vi "菜单-导出py.vi"(8 "error in (no error)":errorcluster caption="错误输入（无错误）", 11 "程序响应 输入":refnum<class "程序响应.lvclass">) -> (0 "error out":errorcluster caption="错误输出", 3 "程序响应 输出":refnum<class "程序响应.lvclass">)   [LabVIEW 2018, in "程序响应.lvlib" / "程序响应.lvclass"]
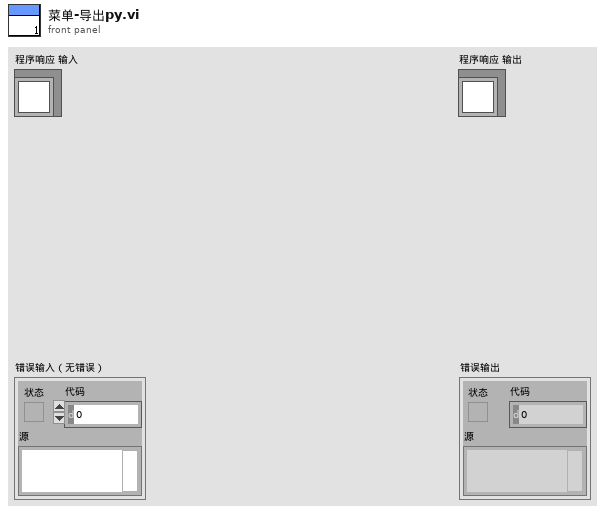
[diagram p1: front panel]
types:
  T1 = enum16{"open", "replace", "create", "open or create", "replace or create", "replace or create with confirmation"}
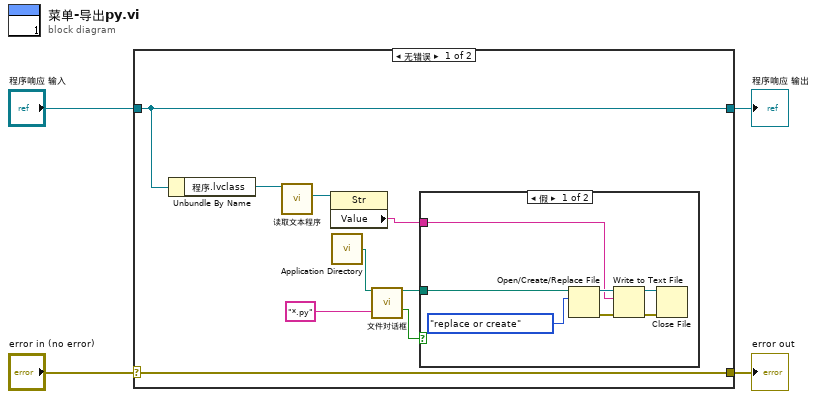
[diagram p0: block diagram]
diagram:
  n1 = case shown="无错误" "error in (no error)" {
    selector: "error in (no error)" -> [w13 w22]
    tunnel: [w13 w22] -> w3
    tunnel: [w12 w21] -> w1
    tunnel: "程序响应 输入" -> [w12 w21]
    frame No Error {
      n2 = Unbundle By Name(w12) -> ("程序.lvclass"=w11:refnum<class "程序.lvclass">)
      n3 = call-dynamic "读取文本程序.vi"("程序输入"=w11) -> ("文本程序"=w10:refnum<vi>)  [unwired: 8 in, 2 out]
      n4 = property class="Str"(reference=w10) -> ("Value"=w6:string)  [unwired: 1 in, 2 out]
      n5 = call <vilib>:"Application Directory.vi"() -> ("Application Directory"=w7:path)
      n6 = call "文件对话框"("start path"=w7, "pattern (all files)"="*.py") -> ("selected path"=w9:path, "cancelled"=w8:bool)  [unwired: 10 in, 2 out]
      n7 = case shown="假" w8 {
        tunnel: w9 -> [w15 _]
        tunnel: w6 -> [w14 _]
        frame False {
          n8 = Open/Create/Replace File(file path (use dialog)=w15, operation (0:open)=T1."replace or create" ("操作(0:open)")) -> (refnum out=w20:refnum<file>, error out=w19:errorcluster)  [unwired: 4 in, 1 out]
          n9 = Write to Text File(file (use dialog)=w20, text=w14, error in=w19) -> (refnum out=w18:refnum<file>, error out=w17:errorcluster)  [unwired: 1 in, 1 out]
          n10 = Close File(refnum=w18, error in=w17) -> ()  [unwired: 2 out]
        }
        frame True {
        }
      }
    }
    frame Error {
    }
  }
  "error out" <- w3
  "程序响应 输出" <- w1
